vi "Level's VI Reference.vi"(1 "Level":i32) -> (0 "Level's VI Reference":refnum<vi>)   [LabVIEW 2012, in "VIRef.lvlib"]
doc: "Returns a reference to the VI at Level."
uses:
  VIRef.lvlib
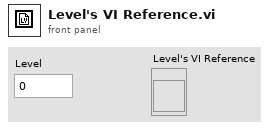
[diagram p1: front panel]
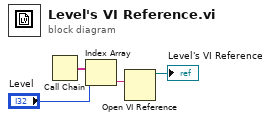
[diagram p0: block diagram]
diagram:
  n1 = Call Chain() -> (call chain=w3:string[])
  n2 = Index Array(array=w3, index="Level") -> (element=w2:string)
  n3 = Open VI Reference(vi path=w2) -> (vi reference=→"Level's VI Reference":refnum<vi>)  [unwired: 5 in, 1 out]
